vi "delete PID from configuration.vi"(8 "error in":errorcluster, 10 "PID In":T1={"ID"="", "Setpoint"=refnum, "Process Variable"=refnum, "Output"=refnum, "PID gains"={"proportional gain (Kc)"=1.0, "integral time (Ti, min)"=0.01, "derivative time (Td, min)"=0.0}, "output range"={"output high"=100.0, "output low"=-100.0}} {"output range"."output low" format="%.2f"; "output range"."output high" format="%.2f"}, 11 "Tagbus PID Module configuration in":refnum<class "Tagbus PID Module configuration.lvclass">) -> (0 "error out":errorcluster, 3 "Tagbus PID Module configuration out":refnum<class "Tagbus PID Module configuration.lvclass">)   [LabVIEW 2014, in "Tagbus PID Module configuration.lvclass"]
doc: "This VI removes the specified VI from the Module Configuration."
uses:
  Tagbus PID Module configuration.lvclass
  <vilib>/NI/Tag Bus Module Framework/channel/TBM channel.lvclass
  Tagbus PID Module configuration.lvclass/Tagbus PID Module configuration.ctl
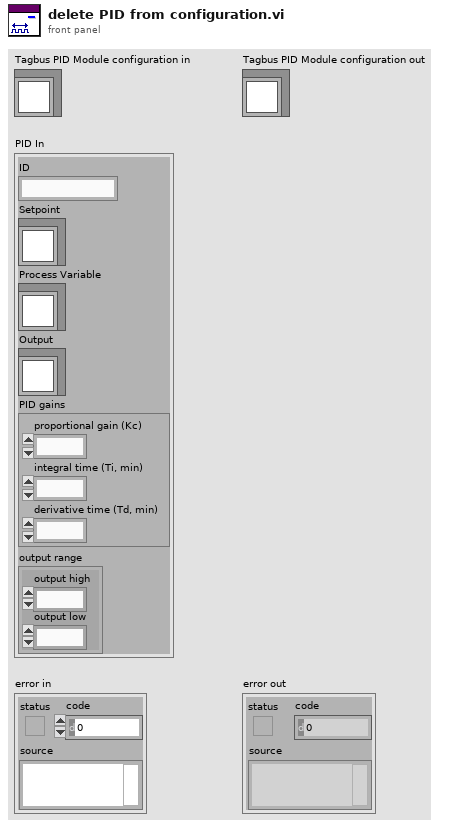
[diagram p1: front panel]
types:
  T1 = cluster{"ID":string, "Setpoint":refnum<class "TBM channel.lvclass">, "Process Variable":refnum<class "TBM channel.lvclass">, "Output":refnum<class "TBM channel.lvclass">, "PID gains":cluster{"proportional gain (Kc)":dbl, "integral time (Ti, min)":dbl, "derivative time (Td, min)":dbl}, "output range":cluster{"output high":dbl, "output low":dbl}}
  T2 = cluster{"ID":string, "Setpoint":refnum<class "TBM channel.lvclass">, "Process Variable":refnum<class "TBM channel.lvclass">, "Output":refnum<class "TBM channel.lvclass">, "PID gains":cluster{"proportional gain (Kc)":dbl, "integral time (Ti, min)":dbl, "derivative time (Td, min)":dbl}, "output range":cluster{"output high":dbl, "output low":dbl}}[]
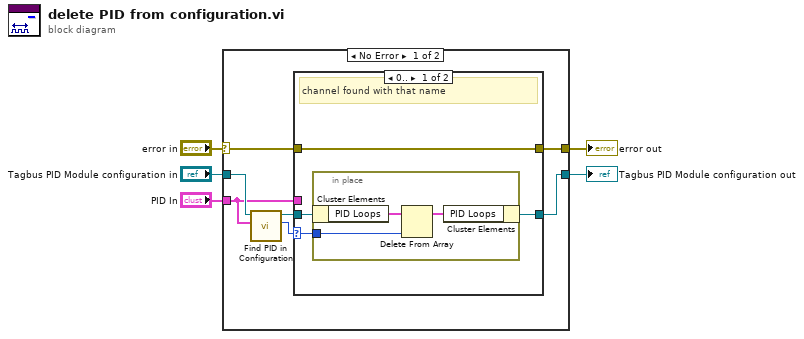
[diagram p0: block diagram]
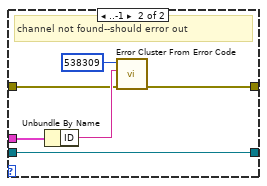
[diagram p2: hidden frame]
diagram:
  n1 = case shown="No Error" "error in" {
    selector: "error in" -> [w7 w26]
    tunnel: "PID In" -> [w6 _]
    tunnel: [w12 w26] -> w5
    tunnel: [w8 w27] -> w4
    tunnel: "Tagbus PID Module configuration in" -> [w11 w27]
    frame No Error {
      n2 = call "Find PID in Configuration.vi"("Channels"=w6, "Tagbus PID Module configuration in"=w11) -> ("index"=w10:i32, "Tagbus PID Module configuration out"=w9:refnum<class "Tagbus PID Module configuration.lvclass">)  [unwired: 8 in]
      n3 = case shown="0.." w10 {
        selector: w10 -> [w16 _]
        tunnel: [w13 w25] -> w12
        tunnel: [w15 w20] -> w8
        tunnel: w9 -> [w14 w20]
        tunnel: w7 -> [w13 w21]
        tunnel: w6 -> [_ w23]
        frame 0.. {
          # "channel found with that name"
          n4 = in-place {
            in-place-border: w16 -> [w19]
            n5 = in-place-cluster #1(w14) -> ("PID Loops"=w17:T2)
            n6 = Delete From Array(array=w17, index=w19) -> (array with subset deleted=w18:T2)  [unwired: 1 in, 1 out]
            n7 = in-place-cluster #1("PID Loops"=w18) -> (w15:refnum<class "Tagbus PID Module configuration.lvclass">)
          }
        }
        frame ..-1 {
          # "channel not found--should error out"
          n8 = Unbundle By Name(w23) -> ("ID"=w22:string)
          n9 = call <vilib>:"Error Cluster From Error Code.vi"("error in (no error)"=w21, "error message (\"\")"=w22, "error code (0)"=538309) -> ("error out"=w25:errorcluster)  [unwired: 6 in]
        }
      }
    }
    frame Error {
    }
  }
  "error out" <- w5
  "Tagbus PID Module configuration out" <- w4
